vi "DAQ6363_ProcRateDat.vi"(0 "Rate Data":i32[][](array[numeric]), 1 "ClearRef":refnum<vi>, 3 "Avg ref":refnum<vi>, 5 "Count Rates":i32[](array[numeric]), 9 "RateAvg Data":i32[][](array[numeric]), 11 "error in (no error)":errorcluster caption="entrée d'erreur (pas d'erreur)", 12 "Avg Val":i32) -> (4 "Rate Data Out":i32[][](array[numeric]), 6 "Data":cluster{dbl, dbl, dbl, dbl}[](array[cluster]), 10 "RateAvg Data Out":i32[][](array[numeric]) format="%.2f", 13 "ValAvg":i32[](array[numeric]), 14 "Avg Val Out":i32, 15 "error out":errorcluster caption="sortie d'erreur")   [LabVIEW 2019]
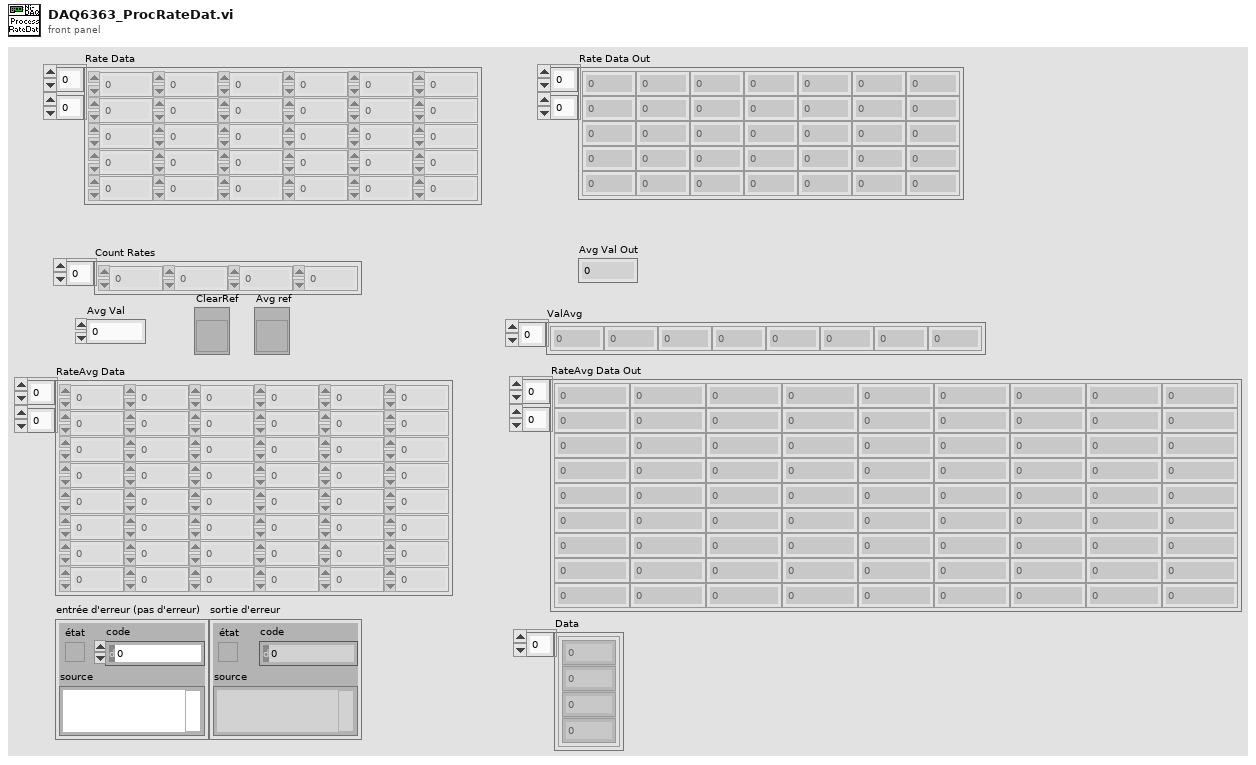
[diagram p1: front panel]
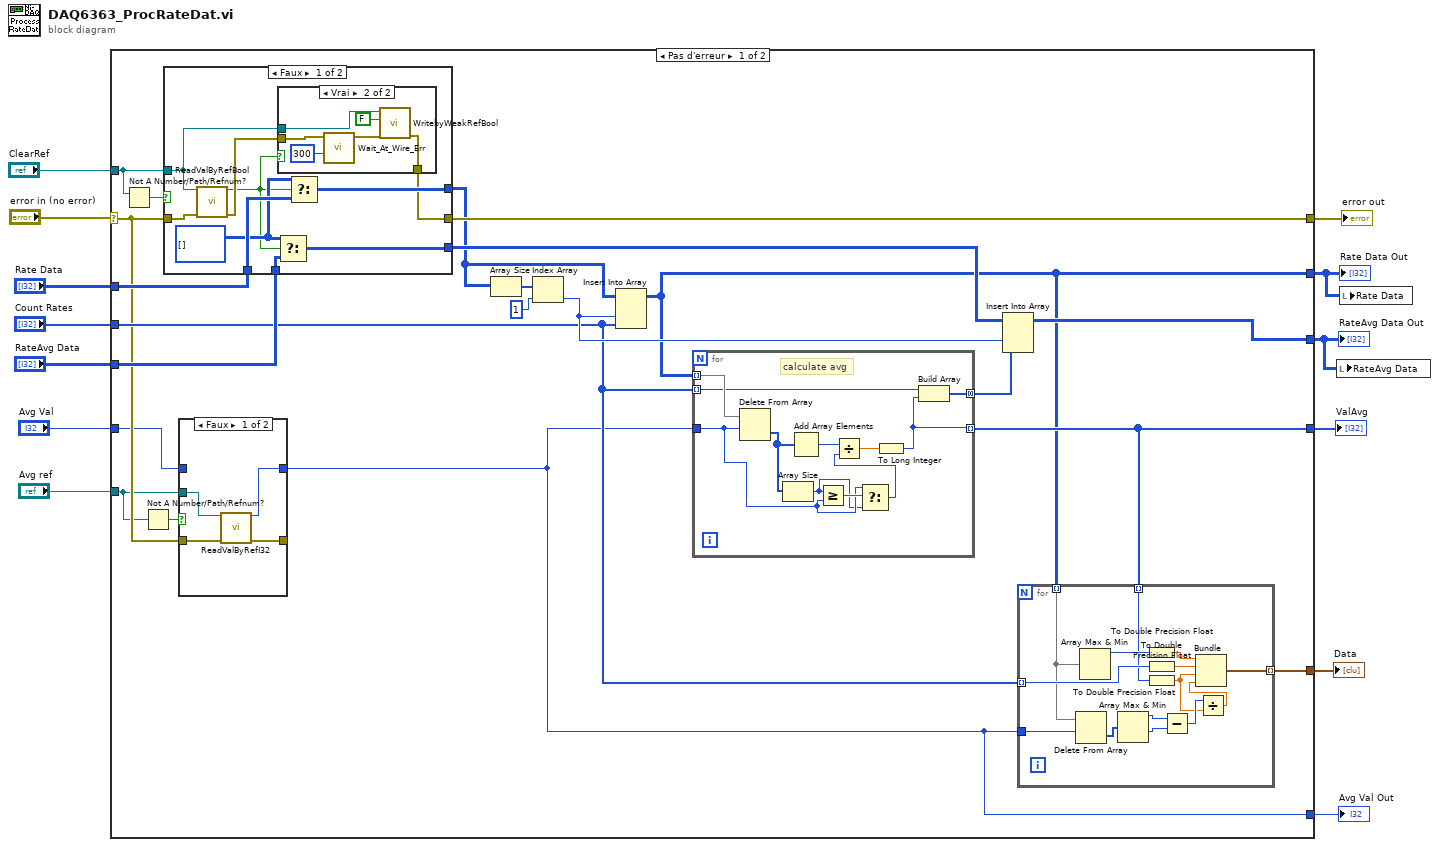
[diagram p0: block diagram]
diagram:
  n1 = case shown="Pas d'erreur" "error in (no error)" {
    selector: "error in (no error)" -> [w21 w88]
    tunnel: "Avg Val" -> [w18 _]
    tunnel: [w16 w87] -> w2
    tunnel: "Rate Data" -> [w26 w87]
    tunnel: "Count Rates" -> [w23 _]
    tunnel: "RateAvg Data" -> [w27 w86]
    tunnel: [w22 w86] -> w1
    tunnel: [w17 _] -> w9
    tunnel: [w30 w88] -> w7
    tunnel: "ClearRef" -> [w28 _]
    tunnel: "Avg ref" -> [w20 _]
    tunnel: [w15 _] -> w4
    tunnel: [w14 _] -> w3
    frame No Error {
      n2 = Not A Number/Path/Refnum?(number/path/refnum=w28) -> (NaN/Path/Refnum?=w29:bool)
      n3 = Not A Number/Path/Refnum?(number/path/refnum=w20) -> (NaN/Path/Refnum?=w19:bool)
      n4 = case shown="Faux" w29 {
        tunnel: w21 -> [w50 w60]
        tunnel: [w43 w60] -> w30
        tunnel: w28 -> [w44 _]
        tunnel: w27 -> [w48 w59]
        tunnel: w26 -> [w49 w58]
        tunnel: [w47 w59] -> w25
        tunnel: [w46 w58] -> w24
        frame False {
          w45 = i32[][] [] ("cas vrai")
          n5 = call <userlib>:"ReadValByRefBool.vi"("Control Ref"=w44, "error in"=w50) -> ("Valeur"=w41:bool, "error out"=w42:errorcluster)  [unwired: 12 in]
          n6 = case shown="Vrai" w41 {
            tunnel: w44 -> [_ w57]
            tunnel: [w51 w56] -> w43
            tunnel: w42 -> [w51 w54]
            frame False {
            }
            frame True {
              n7 = call <userlib>:"Wait_At_Wire_Err.vi"("Wait (ms)"=u32 300, "error in (no error)"=w54) -> ("error out"=w53:errorcluster)  [unwired: 7 in, 2 out]
              n8 = call <userlib>:"WritebyWeakRefBool.vi"("error in"=w53, "Valeur"=FALSE, "Control Ref"=w57) -> ("error out"=w56:errorcluster)  [unwired: 8 in]
            }
          }
          n9 = Select(t=w45, s=w41, f=w48) -> (s? t:f=w47:i32[][])
          n10 = Select(t=w45, s=w41, f=w49) -> (s? t:f=w46:i32[][])
        }
        frame True {
        }
      }
      n11 = case shown="Faux" w19 {
        tunnel: w21 -> [w38 w40]
        tunnel: [w36 w40] -> _
        tunnel: w20 -> [w37 _]
        tunnel: w18 -> [_ w39]
        tunnel: [w35 w39] -> w14
        frame False {
          n12 = call <userlib>:"ReadValByRefI32.vi"("Control Ref"=w37, "error in"=w38) -> ("Valeur"=w35:i32, "error out"=w36:errorcluster)  [unwired: 12 in]
        }
        frame True {
        }
      }
      n13 = Array Size(array=w24) -> (size(s)=w34:i32[])
      n14 = Index Array(array=w34, index=1 ("indice")) -> (element=w32:i32)
      n15 = Insert Into Array(array=w24, index (col)=w32, new element=w23) -> (w16:i32[][])  [unwired: 1 in]
      n16 = for {
        tunnel: w16 -> [w85] mode=indexing
        tunnel: w14 -> [w78]
        tunnel: w23 -> [w82] mode=indexing
        tunnel: [w81] -> w31 mode=concatenating
        tunnel: [w75] -> w17 mode=indexing
        # "calculate avg"
        n17 = Delete From Array(array=w85, length=w78) -> (deleted portion=w80:i32[])  [unwired: 1 in, 1 out]
        n18 = Array Size(array=w80) -> (size(s)=w76:i32)
        n19 = Add Array Elements(numeric array=w80) -> (sum=w84:i32)
        n20 = Greater Or Equal?(x=w76, y=w78) -> (x >= y?=w79:bool)
        n21 = Select(t=w78, s=w79, f=w76) -> (s? t:f=w77:i32)
        n22 = Divide(x=w84, y=w77) -> (x/y=w83:dbl)
        n23 = To Long Integer(number=w83) -> (32bit integer=w75:i32)
        n24 = Build Array(w82, w75) -> (w81:i32[])
      }
      n25 = Insert Into Array(array=w25, index (col)=w32, new element=w31) -> (w22:i32[][])  [unwired: 1 in]
      n26 = for {
        tunnel: w16 -> [w69] mode=indexing
        tunnel: w23 -> [w71] mode=indexing
        tunnel: [w74] -> w15 mode=indexing
        tunnel: w14 -> [w68]
        tunnel: w17 -> [w61] mode=indexing
        n27 = Delete From Array(array=w69, length=w68) -> (deleted portion=w67:i32[])  [unwired: 1 in, 1 out]
        n28 = Array Max & Min(array=w69) -> (max value=w70:i32)  [unwired: 3 out]
        n29 = Array Max & Min(array=w67) -> (max value=w66:i32, min value=w65:i32)  [unwired: 2 out]
        n30 = To Double Precision Float(number=w70) -> (double precision float=w73:dbl)
        n31 = To Double Precision Float(number=w71) -> (double precision float=w72:dbl)
        n32 = To Double Precision Float(number=w61) -> (double precision float=w63:dbl)
        n33 = Subtract(x=w66, y=w65) -> (x-y=w64:i32)
        n34 = Divide(x=w64, y=w63) -> (x/y=w62:dbl)
        n35 = Bundle(w73, w72, w63, w62) -> (w74:cluster{dbl, dbl, dbl, dbl})  [unwired: 1 in]
      }
    }
    frame Error {
    }
  }
  "Rate Data Out" <- w2
  "RateAvg Data Out" <- w1
  "ValAvg" <- w9
  "error out" <- w7
  "Avg Val Out" <- w3
  "Data" <- w4
  n36 = local write "RateAvg Data"(w1) -> ()
  n37 = local write "Rate Data"(w2) -> ()
